vi "load_and_display_SLM.vi"(8 "error in (no error)":errorcluster, 10 "Image Data":u8[][](array[numeric]), 11 "SLM ID":T1) -> (0 "error out":errorcluster, 2 "2D Picture":picture)   [LabVIEW 2025]
uses:
  9a23a187-f6c1-45f4-bcbe-505f61ba8c1f.vi
  <userlib>/HOLOEYE SLM Display SDK 4.1.0/types/heds_slm_id_typedef.ctl
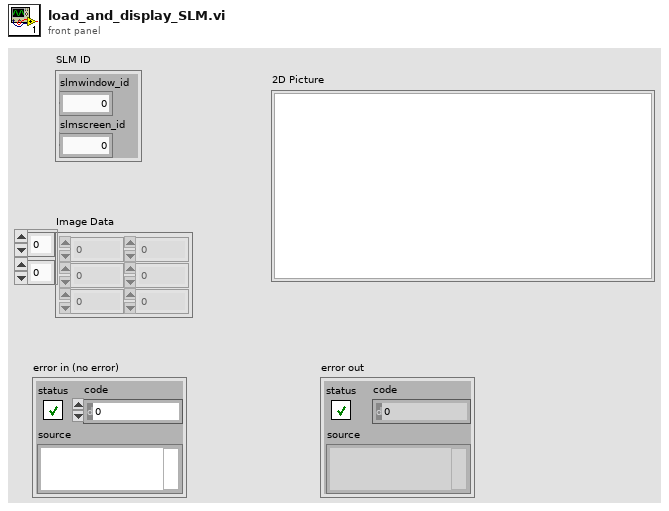
[diagram p1: front panel]
types:
  T1 = typedef "heds_slm_id_typedef.ctl" = cluster{"slmwindow_id":u32, "slmscreen_id":u32}
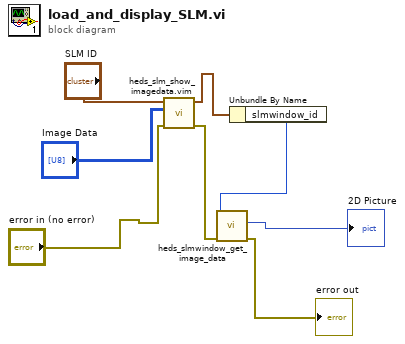
[diagram p0: block diagram]
diagram:
  n1 = call "heds_slm_show_imagedata.vim"("error in (no error)"="error in (no error)", "Image Data"="Image Data", "SLM ID"="SLM ID") -> ("error out"=w1:errorcluster, "SLM ID out"=w7:T1)  [unwired: 6 in, 1 out]
  n2 = Unbundle By Name(w7) -> ("slmwindow_id"=w8:u32)
  n3 = call <userlib>:"heds_slmwindow_get_image_data.vi"("error in (no error)"=w1, "slmwindow_id"=w8) -> ("error out"=→"error out":errorcluster, "2D Picture"=→"2D Picture":picture)  [unwired: 6 in, 2 out]
